vi "Questionable Event Enable.vi"(0 "VISA resource name":refnum<visa-resource-name>, 5 "Questionable Event Enable":T1, 11 "error in (no error)":errorcluster) -> (4 "VISA resource name out":refnum<visa-resource-name>, 15 "error out":errorcluster)   [LabVIEW 2020, in "NH Research Regenerative Test Series.lvlib"]
doc: "Sets the value of the Questionable Enable register. This register is a mask for enabling specific bits from the Questionable Event register to set the questionable summary (QUES) bit of the Status Byte register. This bit (bit 3) is the logical OR of all the Questionable Event register bits that are enabled by the Questionable Status Enable register.\n\nThe Questionable Event Enable consists of the following 15 bits:\n\nBit 0: Reserved\nBit 1: Reserved\nBit 2: Reserved \nBit 3: Reserved\nBit 4: Reserved\nBit 5: Reserved \nBit 6: Reserved\nBit 7: Reserved\nBit 8: Calibration checksum error\nBit 9: Firmware checksum error\nBit 10: Program executing from flash\nBit 11: Installed flash not detected or incorrect\nBit 12: Reserved\nBit 13: Reserved\nBit 14: Reserved"
uses:
  NH Research Regenerative Test Series.lvlib
panel:
  # "Bit 0:  Reserved\nBit 1:  Reserved\nBit 2:  Reserved\t\nBit 3:  Reserved\nBit 4:\t\tReserved\nBit 5:  Reserved\t\nBit 6:  Reserved\nBit 7:  Reserved\nBit 8:  Calibration checksum error\nBit 9:  Firmware checksum error\nBit 10:  Program executing from flash\nBit 11:  Installed flash not detect or incorrect \nBit 12:  Reserved\nBit 13:  Reserved\nBit 14:  Reserved"
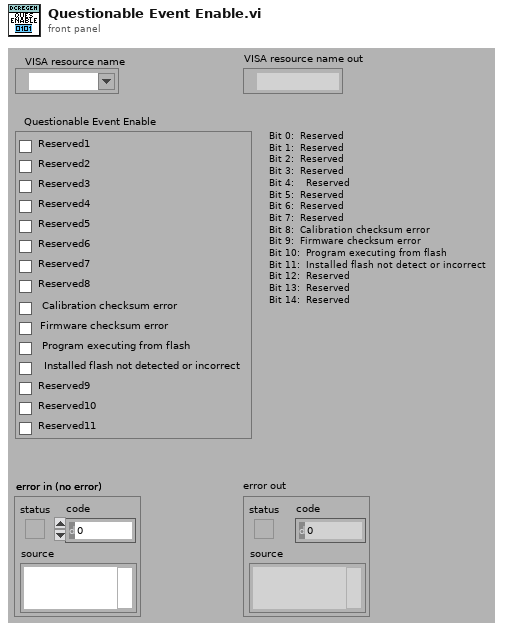
[diagram p1: front panel]
types:
  T1 = cluster{"Reserved1":bool, "Reserved2":bool, "Reserved3":bool, "Reserved4":bool, "Reserved5":bool, "Reserved6":bool, "Reserved7":bool, "Reserved8":bool, "Calibration checksum error":bool, "Firmware checksum error":bool, "Program executing from flash":bool, "Installed flash not detected or incorrect ":bool, "Reserved9":bool, "Reserved10":bool, "Reserved11":bool}
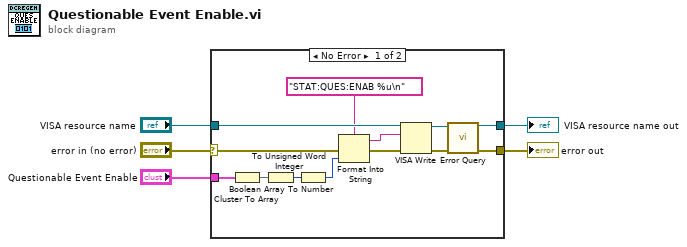
[diagram p0: block diagram]
diagram:
  n1 = case shown="No Error" "error in (no error)" {
    selector: "error in (no error)" -> [w12 w20]
    tunnel: "VISA resource name" -> [w18 w19]
    tunnel: [w16 w19] -> w5
    tunnel: [w14 w20] -> w4
    tunnel: "Questionable Event Enable" -> [w8 _]
    frame No Error {
      n2 = Cluster To Array(cluster=w8) -> (array=w9:bool[])
      n3 = Boolean Array To Number(Boolean array=w9) -> (number=w7:u32)
      n4 = To Unsigned Word Integer(number=w7) -> (unsigned 16bit integer=w6:u16)
      n5 = Format Into String(format string="STAT:QUES:ENAB %u\n" ("Command to Send"), error in=w12, w6) -> (resulting string=w13:string, error out=w11:errorcluster)  [unwired: 1 in]
      n6 = VISA Write(VISA resource name=w18, write buffer=w13, error in (no error)=w11) -> (VISA resource name out=w17:refnum<visa-resource-name>, error out=w15:errorcluster)  [unwired: 1 out]
      n7 = call "Error Query.vi"("VISA resource name"=w17, "error in (no error)"=w15) -> ("VISA resource name out"=w16:refnum<visa-resource-name>, "error out"=w14:errorcluster)  [unwired: 10 in, 2 out]
    }
    frame Error {
    }
  }
  "error out" <- w4
  "VISA resource name out" <- w5
